vi "Write File.vi"(11 "Game Board in":refnum<class "Game Board.lvclass">) -> ()   [LabVIEW 2024, in "Game Board.lvclass"]
doc: "MIT Licence\nCopyright (c) 2024 David Grollier"
uses:
  Game Board.lvclass
  Game Board.lvclass/Game Board.ctl
  Game Board Component/Movable/Movable.lvclass
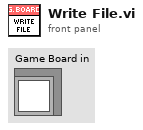
[diagram p1: front panel]
types:
  T1 = enum16{"open", "replace", "create", "open or create", "replace or create", "replace or create with confirmation"}
  T2 = map{string, refnum<class "Game Board Component.lvclass">}
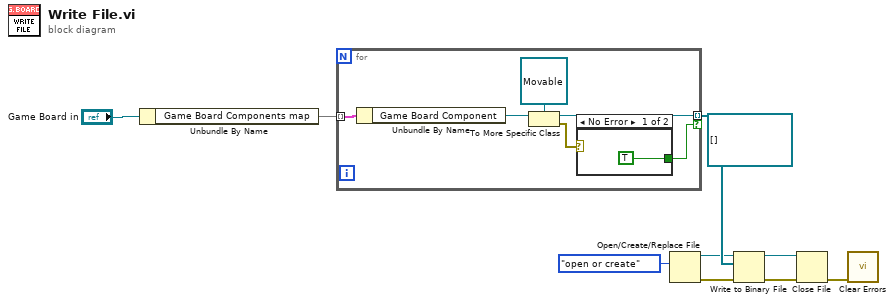
[diagram p0: block diagram]
diagram:
  (unwired) refnum<class "Movable.lvclass">[] []
  n1 = Unbundle By Name("Game Board in") -> ("Game Board Components map"=w9:T2)
  n2 = for {
    tunnel: w9 -> [w14] mode=indexing
    tunnel: [w11] -> w7 mode=indexing if=w10
    n3 = Unbundle By Name(w14) -> ("Game Board Component"=w13:refnum<class "Game Board Component.lvclass">)
    n4 = To More Specific Class(target class=refnum<class "Movable.lvclass"> refnum ("Movable in"), reference=w13) -> (specific class reference=w11:refnum<class "Movable.lvclass">, error out=w12:errorcluster)  [unwired: 1 in]
    n5 = case shown="No Error" w12 {
      tunnel: [TRUE _] -> w10
      frame No Error {
      }
      frame Error {
      }
    }
  }
  n6 = Open/Create/Replace File(operation (0:open)=T1."open or create") -> (refnum out=w6:refnum<file>, error out=w3:errorcluster)  [unwired: 5 in, 1 out]
  n7 = Write to Binary File(file (use dialog)=w6, data=w7, error in=w3) -> (refnum out=w5:refnum<file>, error out=w4:errorcluster)  [unwired: 3 in, 1 out]
  n8 = Close File(refnum=w5, error in=w4) -> (error out=w1:errorcluster)  [unwired: 1 out]
  n9 = call <vilib>:"Clear Errors.vi"("error in (no error)"=w1) -> ()  [unwired: 5 in, 2 out]
